vi "dfd_Multirate Filter Check Order.vi"(7 "zeroPhase?":bool=TRUE, 8 "error in (no error)":errorcluster, 11 "order":i32=20) -> (0 "error out":errorcluster, 3 "dup order":i32=20)   [LabVIEW 2017, in "NI_DigFilter_Process.lvlib"]
uses:
  <vilib>/addons/Digital Filter Design/NI_DigFilter_Process.lvlib
  <vilib>/addons/Digital Filter Design/_Misc.llb/dfd_Error Handlers (Single).vi
  <vilib>/addons/Digital Filter Design/NI_DigFilterLicensed.lvlib
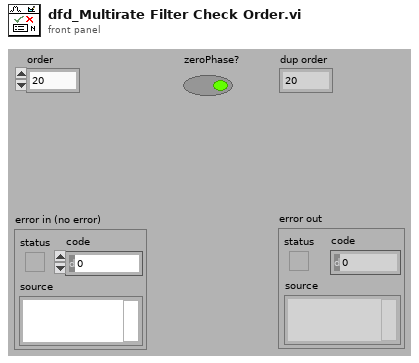
[diagram p1: front panel]
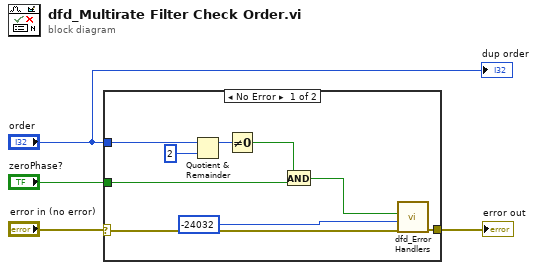
[diagram p0: block diagram]
diagram:
  n1 = case shown="No Error" "error in (no error)" {
    selector: "error in (no error)" -> [w12 w14]
    tunnel: [w13 w14] -> w4
    tunnel: "order" -> [w9 _]
    tunnel: "zeroPhase?" -> [w7 _]
    frame No Error {
      n2 = Quotient & Remainder(x=w9, y=2) -> (x-y*floor(x/y)=w10:i32)  [unwired: 1 out]
      n3 = Not Equal To 0?(x=w10) -> (x != 0?=w6:bool)
      n4 = And(x=w6, y=w7) -> (x .and. y?=w5:bool)
      n5 = call-poly <vilib>:"dfd_Error Handlers.vi"("error in (no error)"=w12, "error code"=-24032 ("ERR_ORDER_ODD"), "condition failed?"=w5) -> ("error out"=w13:errorcluster)  [unwired: 8 out]
    }
    frame Error {
    }
  }
  "error out" <- w4
  "dup order" <- "order"
